vi "buildArrayMinMaxStep.vi"(8 "max (10)":i32=10, 9 "step (1)":i32=1, 10 "min (0)":i32) -> (1 "array":i32[](array[numeric]))   [LabVIEW 2015, in "Tausand AB1000.lvlib"]
doc: "Builds an array of integer numbers, starting at min, ending at max, with regular increment given by step."
uses:
  <instrlib>/Tausand AB1000/Tausand AB1000.lvlib
panel:
  out "negative step?":bool
  out "desired array size":i32
  out "max-min":i32
  out "actual step":i32
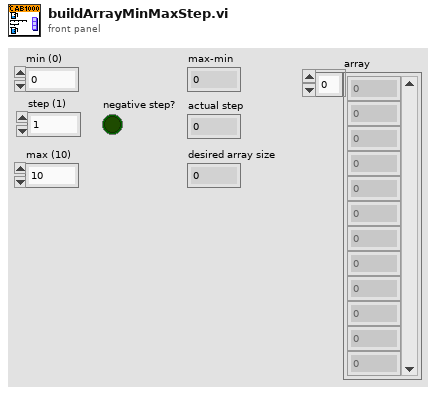
[diagram p1: front panel]
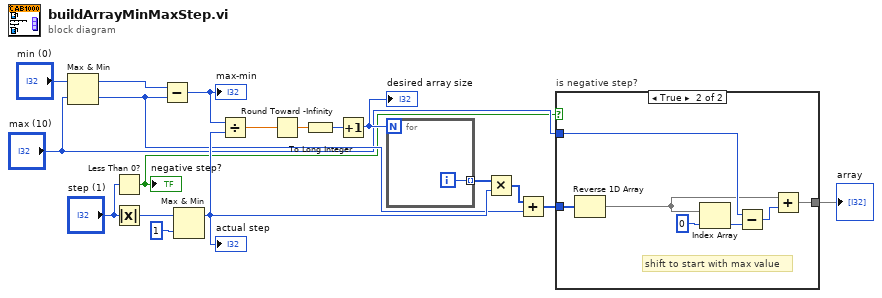
[diagram p0: block diagram]
diagram:
  n1 = Max & Min(x="min (0)", y="max (10)") -> (max(x,y)=w8:i32, min(x,y)=w7:i32)
  n2 = Less Than 0?(x="step (1)") -> (x < 0?=w2:bool)
  "negative step?" <- w2
  n3 = Absolute Value(x="step (1)") -> (abs(x)=w6:i32)
  n4 = Subtract(x=w8, y=w7) -> (x-y=w9:i32)
  "max-min" <- w9
  n5 = Max & Min(x=w6, y=1) -> (max(x,y)=w16:i32)  [unwired: 1 out]
  "actual step" <- w16
  n6 = Divide(x=w9, y=w16) -> (x/y=w17:dbl)
  n7 = Round Toward -Infinity(1:w17) -> (0:w18:dbl)
  n8 = To Long Integer(number=w18) -> (32bit integer=w12:i32)
  n9 = Increment(x=w12) -> (x+1=w11:i32)
  "desired array size" <- w11
  n10 = for {
    N: w11 -> [_]
    tunnel: [w19] -> w13 mode=indexing
    i -> [w19]
  }
  n11 = Multiply(x=w13, y=w16) -> (x*y=w14:i32[])
  n12 = Add(x=w14, y=w7) -> (x+y=w4:i32[])
  n13 = case "is negative step?" shown="True" w2 {
    tunnel: w4 -> [w20 w27]
    tunnel: "max (10)" -> [_ w25]
    tunnel: [w20 w21] -> w1
    frame False {
    }
    frame True {
      # "shift to start with max value"
      n14 = Reverse 1D Array(array=w27) -> (reversed array=w23:i32[])
      n15 = Index Array(array=w23, index=0) -> (element=w24:i32)
      n16 = Subtract(x=w25, y=w24) -> (x-y=w22:i32)
      n17 = Add(x=w23, y=w22) -> (x+y=w21:i32[])
    }
  }
  "array" <- w1
